vi "Get Library Info.vi"(0 "object in":refnum<class "PowerModuleInterface.lvclass">, 11 "Error In":errorcluster) -> (4 "object out":refnum<class "PowerModuleInterface.lvclass">, 6 "PPL Filename":string, 8 "Build Version":string="v1.2.3.4", 15 "Error Out":errorcluster)   [LabVIEW 2023, in "PowerModuleInterface.lvlib" / "PowerModuleInterface.lvclass"]
uses:
  PowerModuleInterface.lvclass
  <vilib>/Utility/LVLibp/NI_PackedLibraryUtility.lvlib
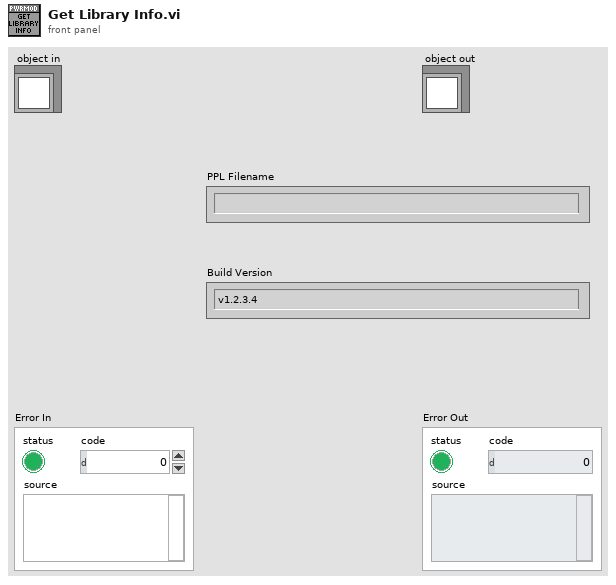
[diagram p1: front panel]
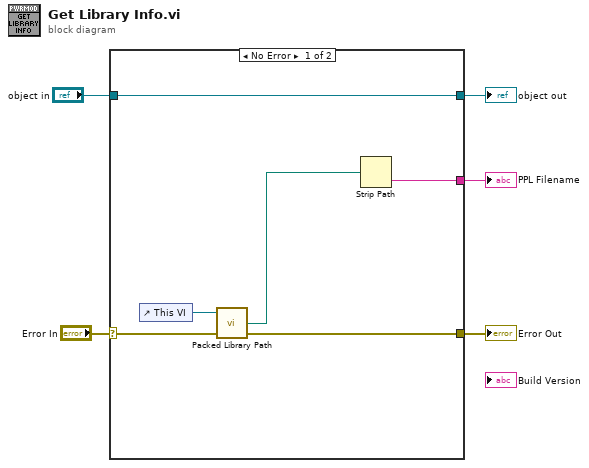
[diagram p0: block diagram]
diagram:
  n1 = case shown="No Error" "Error In" {
    selector: "Error In" -> [w7 w13]
    tunnel: [w6 w13] -> w3
    tunnel: [w11 w12] -> w1
    tunnel: "object in" -> [w11 w12]
    tunnel: [w10 _] -> w2
    frame No Error {
      n2 = control-ref of="This VI"() -> (w8:refnum<vi>)
      n3 = call <vilib>:"Packed Library Path.vi"("error in (no error)"=w7, "vi reference"=w8) -> ("error out"=w6:errorcluster, "packed library path"=w9:path)  [unwired: 1 in, 1 out]
      n4 = Strip Path(path=w9) -> (name=w10:string)  [unwired: 1 out]
    }
    frame Error {
    }
  }
  "Error Out" <- w3
  "object out" <- w1
  "PPL Filename" <- w2
